vi "RightLeft.vi"   [LabVIEW 2017]
types:
  T1 = typedef "Command Status Info.ctl" = cluster{"Name":string, "Status":T2, "notifier out":T3}
  T2 = typedef "Completion Status.ctl" = enum16{"Successful", "Aborted", "Incomplete"}
  T3 = typedef "Completion Notifier.ctl" = refnum<notifier>
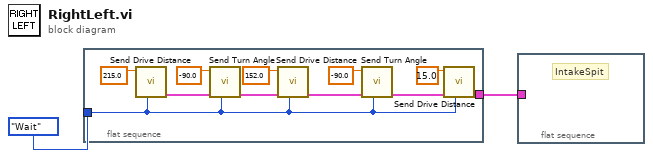
[diagram p0: block diagram]
diagram:
  n1 = flat-sequence {
    tunnel: enum16{"Start", "Wait"}."Wait" ("Synchronization") -> [w4]
    tunnel: [w3] -> w2
    frame #0 {
      n2 = call "Send Drive Distance.vi"("Synchronization"=w4, "Target Distance"=215.0) -> ("Command Info Out"=w8:T1)  [unwired: 8 in, 1 out]
      n3 = call "Send Turn Angle.vi"("Synchronization"=w4, "Command Info In"=w8, "Target Angle"=-90.0) -> ("Command Info Out"=w7:T1)  [unwired: 7 in, 1 out]
      n4 = call "Send Drive Distance.vi"("Synchronization"=w4, "Command Info In"=w7, "Target Distance"=152.0) -> ("Command Info Out"=w6:T1)  [unwired: 7 in, 1 out]
      n5 = call "Send Turn Angle.vi"("Synchronization"=w4, "Command Info In"=w6, "Target Angle"=-90.0) -> ("Command Info Out"=w5:T1)  [unwired: 7 in, 1 out]
      n6 = call "Send Drive Distance.vi"("Synchronization"=w4, "Command Info In"=w5, "Target Distance"=15.0) -> ("Command Info Out"=w3:T1)  [unwired: 7 in, 1 out]
    }
  }
  n7 = flat-sequence {
    tunnel: w2 -> [_]
    frame #0 {
      # "IntakeSpit"
    }
  }
